vi "GamePlayfield_CopyToDraw.vi"(2 "Player":u8) -> ()   [LabVIEW 2018]
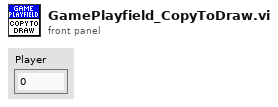
[diagram p1: front panel]
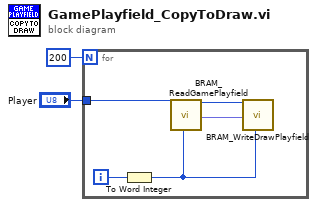
[diagram p0: block diagram]
diagram:
  n1 = for {
    N: 200 -> [_]
    tunnel: "Player" -> [w6]
    i -> [w5]
    n2 = To Word Integer(number=w5) -> (16bit integer=w4:i16)
    n3 = call "BRAM_ReadGamePlayfield.vi"("Player IN"=w6, "Address"=w4) -> ("Player OUT"=w7:u8, "Data"=w3:fxp<+,3,3>)  [unwired: 16 in]
    n4 = call "BRAM_WriteDrawPlayfield.vi"("Player IN"=w7, "Data"=w3, "Address"=w4) -> ()  [unwired: 16 in, 1 out]
  }
